vi "trabalho, terceira aula.vi"() -> (0 "Corrente fase A":dynamicdata(graph), 1 "Tensão fase A":dynamicdata(graph), 2 "Timestamp":dynamicdata(graph), 3 "Corrente fase C":dynamicdata(graph), 4 "Tensão fase C":dynamicdata(graph), 5 "Corrente fase B":dynamicdata(graph), 6 "Tensão fase B":dynamicdata(graph))   [LabVIEW 2024]
panel:
  out "Fase C":string[][](table)
  out "Fase B":string[][](table)
  out "Fase A":string[][](table)
  out "timnestamp":string[][](table)
  out "Waveform Graph":dynamicdata(graph)
  out "All data":string[][](table)
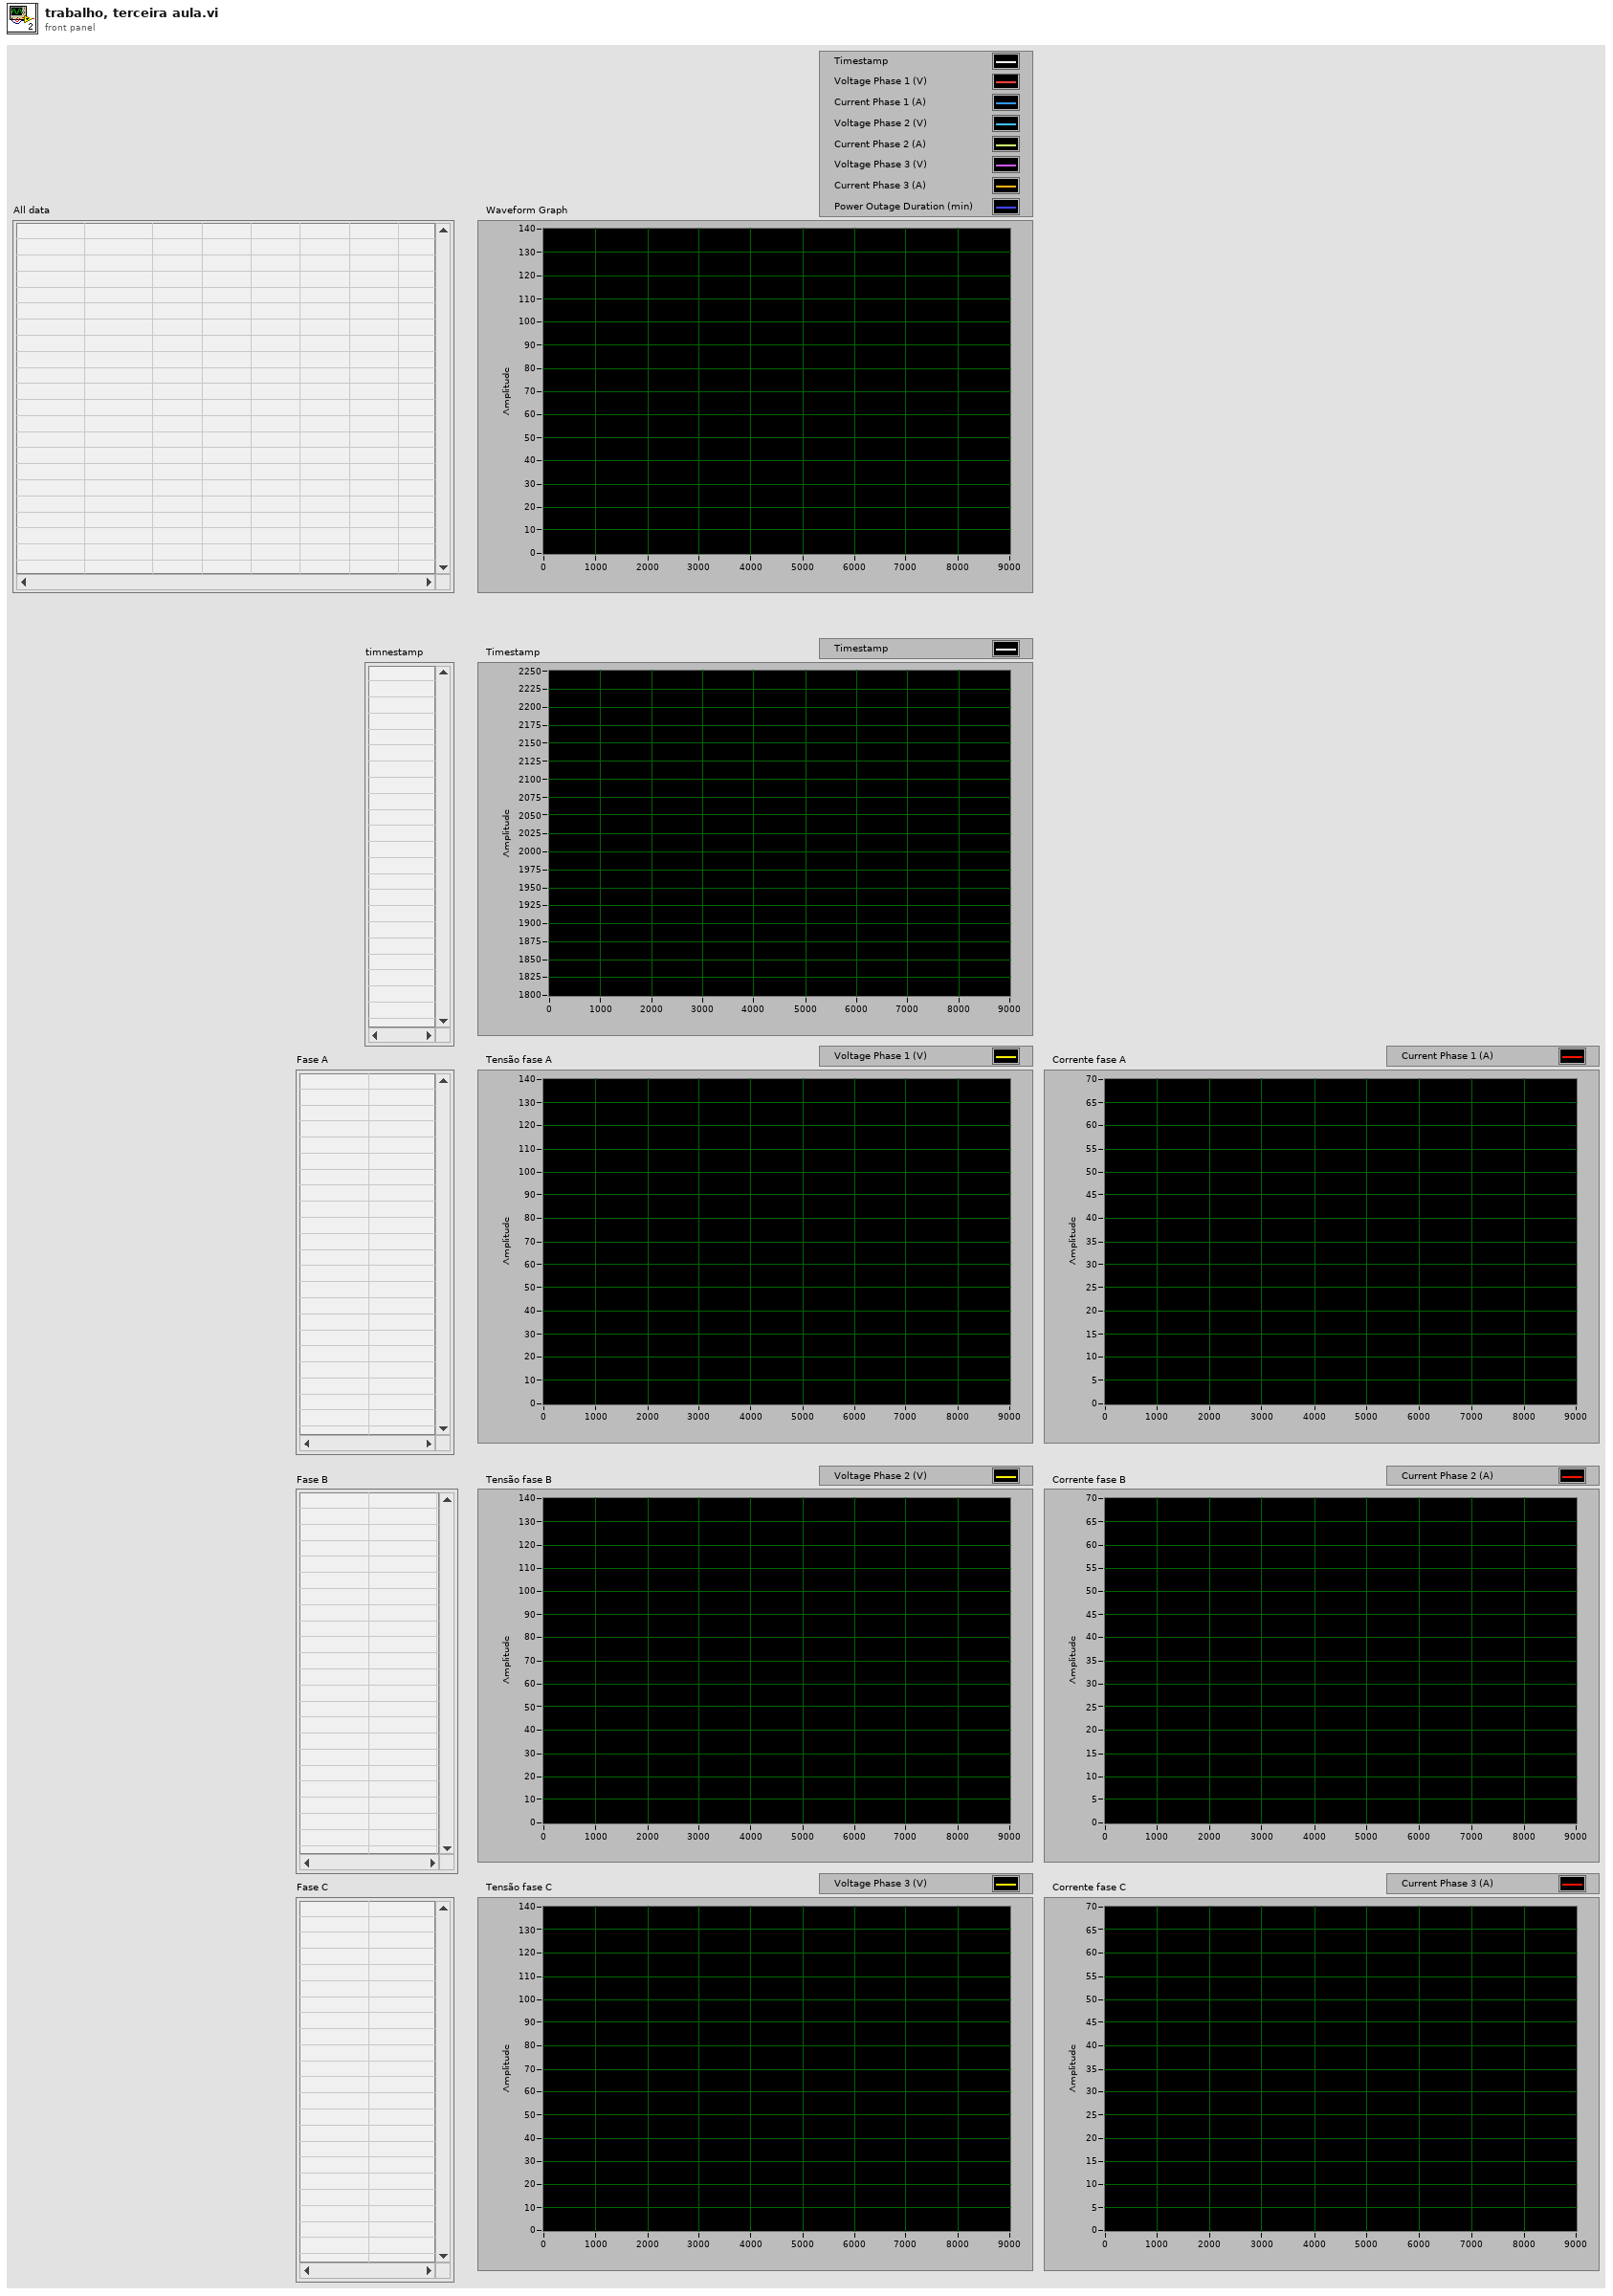
[diagram p1: front panel]
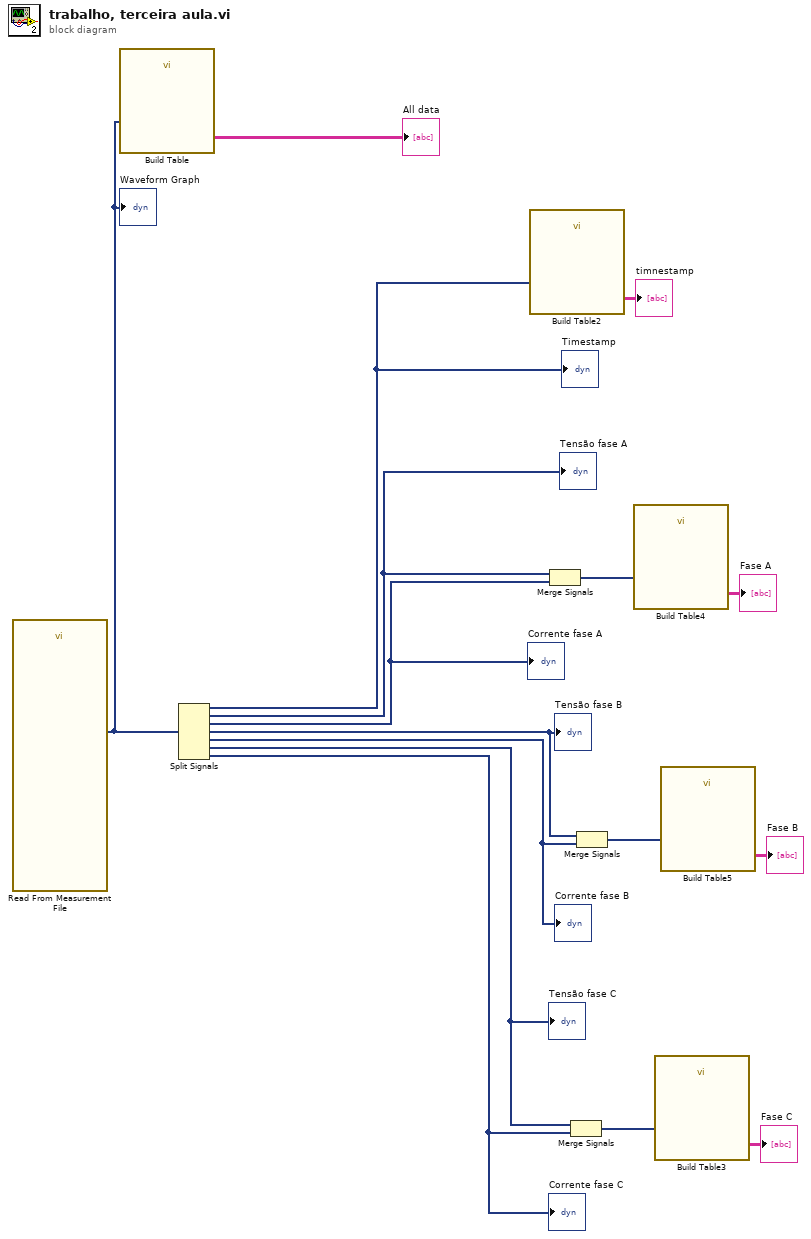
[diagram p0: block diagram]
diagram:
  n1 = call "Read From Measurement File"() -> ("Signals"=w15:dynamicdata)  [unwired: 6 in, 5 out]
  "Waveform Graph" <- w15
  n2 = call "Build Table"("Signals"=w15) -> ("Table"=→"All data":string[][])  [unwired: 4 in, 6 out]
  n3 = Split Signals(w15) -> (w13:dynamicdata, w10:dynamicdata, w8:dynamicdata, w7:dynamicdata, w6:dynamicdata, w2:dynamicdata, w1:dynamicdata)  [unwired: 7 in]
  "Timestamp" <- w13
  "Tensão fase B" <- w7
  "Corrente fase B" <- w6
  "Tensão fase A" <- w10
  "Corrente fase A" <- w8
  "Tensão fase C" <- w2
  "Corrente fase C" <- w1
  n4 = call "Build Table2"("Signals"=w13) -> ("Table"=→"timnestamp":string[][])  [unwired: 4 in, 6 out]
  n5 = Merge Signals(w10, w8) -> (w9:dynamicdata)
  n6 = Merge Signals(w2, w1) -> (w3:dynamicdata)
  n7 = Merge Signals(w7, w6) -> (w5:dynamicdata)
  n8 = call "Build Table4"("Signals"=w9) -> ("Table"=→"Fase A":string[][])  [unwired: 4 in, 6 out]
  n9 = call "Build Table3"("Signals"=w3) -> ("Table"=→"Fase C":string[][])  [unwired: 4 in, 6 out]
  n10 = call "Build Table5"("Signals"=w5) -> ("Table"=→"Fase B":string[][])  [unwired: 4 in, 6 out]
